vi "l_model_forward.vi"(2 "parameters":map{string, dbl[][]}(c390), 3 "X":dbl[][](array[numeric])) -> (0 "caches":T1(array[cluster]), 1 "AL":dbl[][](array[numeric]))   [LabVIEW 2020]
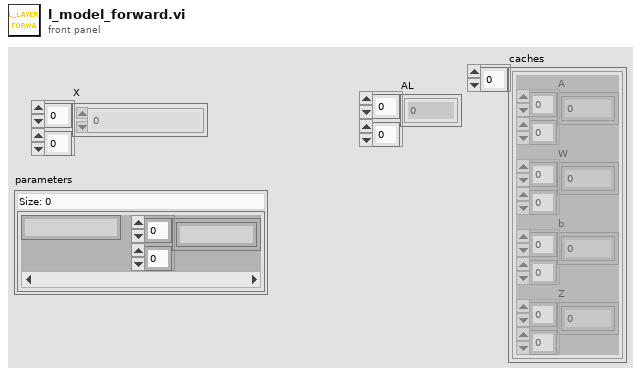
[diagram p1: front panel]
types:
  T1 = cluster{"A":dbl[][], "W":dbl[][], "b":dbl[][], "Z":dbl[][]}[]
  T2 = cluster{"A":dbl[][], "W":dbl[][], "b":dbl[][], "Z":dbl[][]}
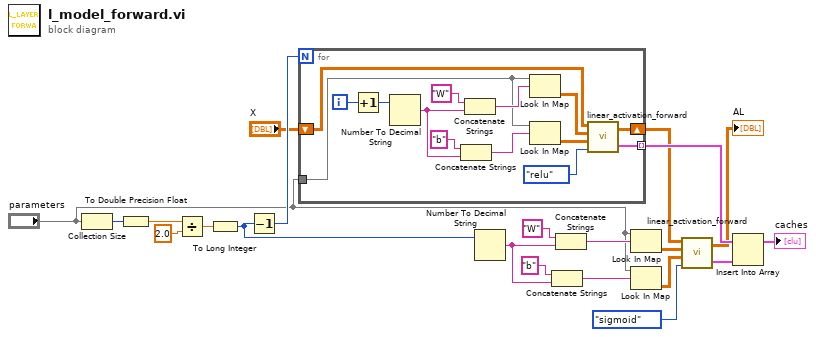
[diagram p0: block diagram]
diagram:
  n1 = Collection Size(1:"parameters") -> (0:w21:i32)
  n2 = To Double Precision Float(number=w21) -> (double precision float=w20:dbl)
  n3 = Divide(x=w20, y=2.0) -> (x/y=w18:dbl)
  n4 = To Long Integer(number=w18) -> (32bit integer=w7:i32)
  n5 = Decrement(x=w7) -> (x-1=w17:i32)
  n6 = for {
    N: w17 -> [_]
    shift-right: [w23] -> w5
    shift-left: "X" -> [w35]
    tunnel: "parameters" -> [w22]
    tunnel: [w24] -> w15 mode=indexing
    i -> [w32]
    n7 = Increment(x=w32) -> (x+1=w31:i32)
    n8 = Number To Decimal String(number=w31) -> (decimal integer string=w27:string)  [unwired: 1 in]
    n9 = Concatenate Strings("b" ("string"), w27) -> (w26:string)
    n10 = Concatenate Strings("W" ("string"), w27) -> (w34:string)
    n11 = Look In Map(map=w22, key=w34) -> (value=w30:dbl[][])  [unwired: 1 in, 1 out]
    n12 = Look In Map(map=w22, key=w26) -> (value=w29:dbl[][])  [unwired: 1 in, 1 out]
    n13 = call "linear_activation_forward.vi"("activation"=enum16{"sigmoid", "relu"}."relu", "b"=w29, "W"=w30, "A_prev"=w35) -> ("cache"=w24:T2, "A"=w23:dbl[][])
  }
  n14 = Number To Decimal String(number=w7) -> (decimal integer string=w13:string)  [unwired: 1 in]
  n15 = Concatenate Strings("b" ("string"), w13) -> (w12:string)
  n16 = Concatenate Strings("W" ("string"), w13) -> (w11:string)
  n17 = Look In Map(map="parameters", key=w11) -> (value=w4:dbl[][])  [unwired: 1 in, 1 out]
  n18 = Look In Map(map="parameters", key=w12) -> (value=w3:dbl[][])  [unwired: 1 in, 1 out]
  n19 = call "linear_activation_forward.vi"("activation"=enum16{"sigmoid", "relu"}."sigmoid", "b"=w3, "W"=w4, "A_prev"=w5) -> ("cache"=w6:T2, "A"=→"AL":dbl[][])
  n20 = Insert Into Array(array=w15, new element=w6) -> (→"caches":T1)  [unwired: 1 in]
